vi "Get Waveform DVRs.vi"(7 "Timeout in (ms)":i32=100, 8 "error in (no error)":errorcluster, 9 "Ignore Read Lock":bool, 10 "Number of Waveforms":i32=2, 11 "DVR Circular Buffer in":refnum<data-value>[](array[refnum])) -> (0 "error out":errorcluster, 1 "Timeout":bool, 2 "DVRs":refnum<data-value>[](array[refnum]), 3 "DVR Circular Buffer out":refnum<data-value>[](array[refnum]), 5 "Remaining timeout (ms)":i32=100)   [LabVIEW 2021, in "CIF_NIChn_DAQ_Base.lvclass"]
uses:
  CIF_NIChn_DAQ_Base.lvclass
  Typedef/Datatype Waveform Channel.ctl
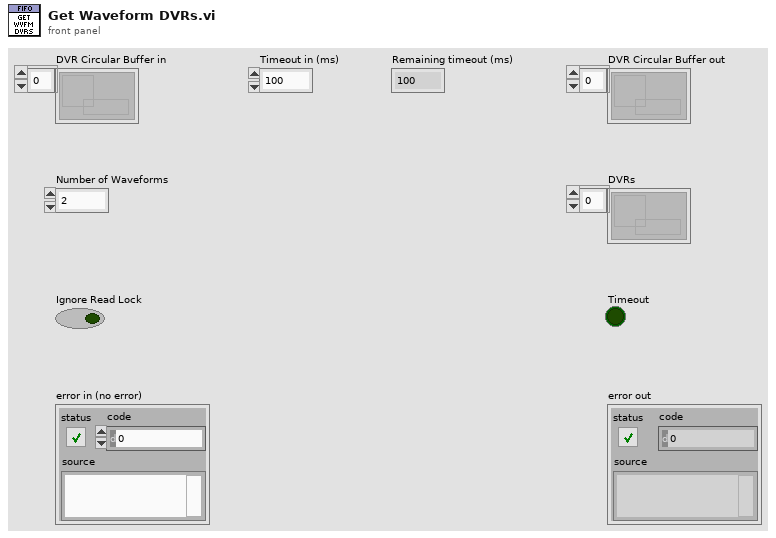
[diagram p1: front panel]
types:
  T1 = typedef "ChannelCommon.lvlib/Datatype Waveform.ctl" = cluster{"measurement":dbl[], "dT":dbl, "Timestamp":i64, "Read Lock":bool}
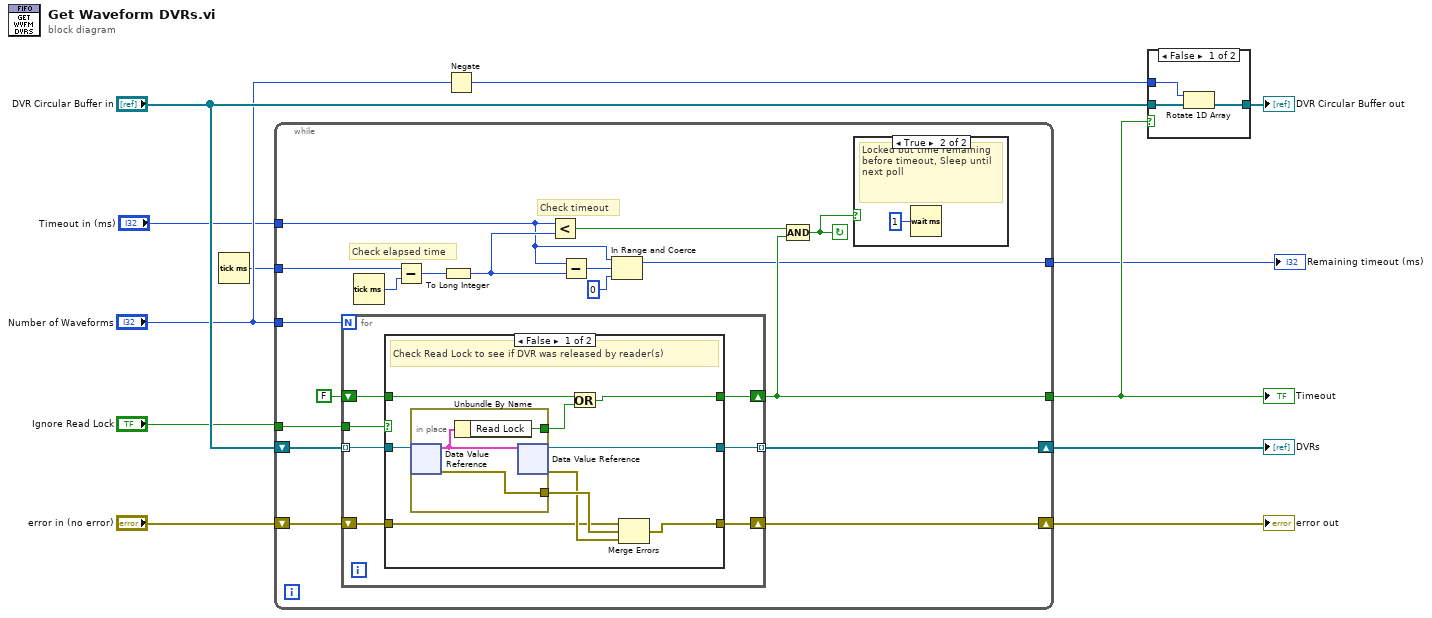
[diagram p0: block diagram]
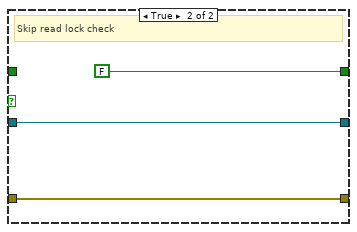
[diagram p3: hidden frame]
diagram:
  n1 = Tick Count (ms)() -> (millisecond timer value=w3:u32)
  n2 = while {
    tunnel: "Number of Waveforms" -> [w25]
    shift-right: [w28] -> w9
    shift-left: "DVR Circular Buffer in" -> [w30]
    shift-right: [w24] -> w5
    shift-left: "error in (no error)" -> [w26]
    tunnel: "Ignore Read Lock" -> [w29]
    tunnel: [w23] -> w4
    tunnel: w3 -> [w22]
    tunnel: "Timeout in (ms)" -> [w13]
    tunnel: [w20] -> w1
    stop <- w21 continue-if-true
    # "Check timeout"
    # "Check elapsed time"
    n3 = for {
      N: w25 -> [_]
      tunnel: w30 -> [w38] mode=indexing
      shift-right: [w34] -> w23
      shift-left: FALSE ("Read Lock") -> [w35]
      tunnel: w29 -> [w37]
      tunnel: [w36] -> w28 mode=indexing
      shift-right: [w32] -> w24
      shift-left: w26 -> [w33]
      n4 = case shown="False" w37 {
        tunnel: w38 -> [w47 w52]
        tunnel: [w44 w52] -> w36
        tunnel: w35 -> [w43 _]
        tunnel: [w41 FALSE ("Read Lock")] -> w34
        tunnel: w33 -> [w40 w51]
        tunnel: [w39 w51] -> w32
        frame False {
          # "Check Read Lock to see if DVR was released by reader(s)"
          n5 = in-place {
            in-place-border: [w50] -> w42
            in-place-border: [w48] -> w46
            n6 = in-place-dvr #1(w47) -> (w49:T1, w48:errorcluster)
            n7 = Unbundle By Name(w49) -> ("Read Lock"=w50:bool)
            n8 = in-place-dvr #1(w49) -> (w44:refnum<data-value>, w45:errorcluster)
          }
          n9 = Or(x=w43, y=w42) -> (x .or. y?=w41:bool)
          n10 = Merge Errors(w40, w46, w45) -> (w39:errorcluster)
        }
        frame True {
          # "Skip read lock check"
        }
      }
    }
    n11 = Tick Count (ms)() -> (millisecond timer value=w19:u32)
    n12 = Subtract(x=w22, y=w19) -> (x-y=w18:u32)
    n13 = To Long Integer(number=w18) -> (32bit integer=w17:i32)
    n14 = Less?(x=w13, y=w17) -> (x < y?=w14:bool)
    n15 = Subtract(x=w13, y=w17) -> (x-y=w16:i32)
    n16 = In Range and Coerce(upper limit=w13, x=w16, lower limit=0) -> (coerced(x)=w20:i32)  [unwired: 1 out]
    n17 = Compound Arithmetic op=AND(w14, w23) -> (w21:bool)
    n18 = case shown="True" w21 {
      frame False {
        # "Exit"
      }
      frame True {
        # "Locked but time remaining before timeout, Sleep until next poll"
        n19 = Wait (ms)(milliseconds to wait=u32 1) -> ()  [unwired: 1 out]
      }
    }
  }
  "Timeout" <- w4
  "error out" <- w5
  "DVRs" <- w9
  "Remaining timeout (ms)" <- w1
  n20 = Negate(x="Number of Waveforms") -> (-x=w6:i32)
  n21 = case shown="False" w4 {
    tunnel: "DVR Circular Buffer in" -> [w56 w57]
    tunnel: [w55 w57] -> w12
    tunnel: w6 -> [w54 _]
    frame False {
      n22 = Rotate 1D Array(1:w56, 2:w54) -> (0:w55:refnum<data-value>[])
    }
    frame True {
    }
  }
  "DVR Circular Buffer out" <- w12
